vi "Nickname (Read).vi"(6 "ISOBUS address":T2=-1 caption="ISOBUS address (-1)", 8 "error in":errorcluster, 11 "Mercury Reference In":T3) -> (0 "error out":errorcluster, 2 "Nickname":string, 3 "Mercury Reference Out":T3, 4 "Valid?":T1)   [LabVIEW 2013, in "Mercury iXX.lvlib" / "Pressure.lvlib"]
doc: "Read the Nickname of the selected pressure device."
uses:
  <instrlib>/Mercury iXX/Public/Libraries/Pressure.lvlib
  <instrlib>/Mercury iXX/Public/Controls/Mercury Reference.ctl
  <instrlib>/Mercury iXX/Public/Controls/Comms Transport Layer.ctl
  <instrlib>/Mercury iXX/Private/Controls/Query Dynamic Reference.ctl
  <instrlib>/Mercury iXX/Public/Controls/ISOBus Address.ctl
  <instrlib>/Mercury iXX/Public/Controls/Is Valid LED.ctl
  <instrlib>/Mercury iXX/Private/Controls/Command Verbs.ctl
  <instrlib>/Mercury iXX/Mercury iXX.lvlib
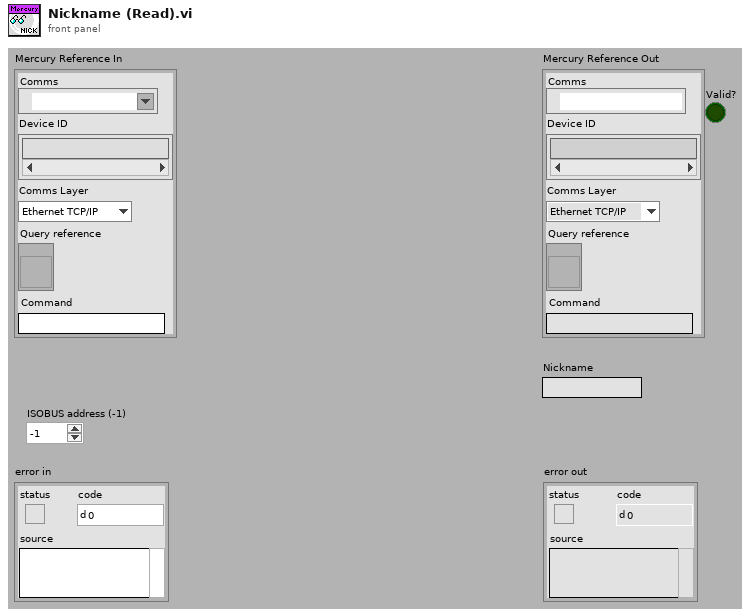
[diagram p1: front panel]
types:
  T1 = typedef "Mercury iXX.lvlib/Is Valid LED.ctl" = bool
  T2 = typedef "Mercury iXX.lvlib/ISOBus Address.ctl" = i32
  T3 = typedef "Mercury iXX.lvlib/Mercury Reference.ctl" = cluster{"Comms":refnum<visa-resource-name>, "Device ID":string[], "Comms Layer":T4, "Command":string, "Query reference":T5}
  T4 = typedef "Mercury iXX.lvlib/Comms Transport Layer.ctl" = enum16{"Ethernet TCP/IP", "USB", "ISOBus - RS-232", "GPIB"}
  T5 = typedef "Mercury iXX.lvlib/Query Dynamic Reference.ctl" = refnum<vi>
  T6 = typedef "Mercury iXX.lvlib/Command Verbs.ctl" = string
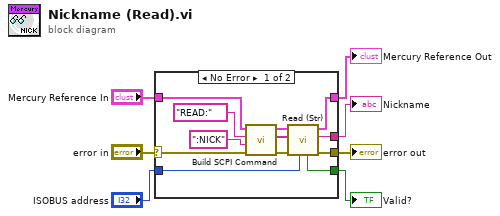
[diagram p0: block diagram]
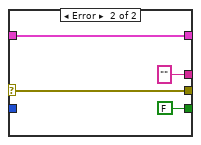
[diagram p2: hidden frame]
diagram:
  n1 = case shown="No Error" "error in" {
    selector: "error in" -> [w8 w23]
    tunnel: [w14 w22] -> w7
    tunnel: "Mercury Reference In" -> [w13 w22]
    tunnel: "ISOBUS address" -> [w12 _]
    tunnel: [w11 T1 FALSE ("Valid?")] -> w4
    tunnel: [w10 w23] -> w3
    tunnel: [w9 "" ("Response")] -> w2
    frame No Error {
      n2 = call <instrlib>:"Build SCPI Command.vi"("error in"=w8, "Noun(s)"=":NICK" ("Command"), "Verb"=T6 "READ:", "Mercury Reference In"=w13) -> ("error out"=w19:errorcluster, "SCPI Message(s)"=w16:string[], "Mercury Reference Out"=w17:T3)  [unwired: 5 out]
      n3 = call <instrlib>:"Read (Str).vi"("ISOBUS address"=w12, "error in"=w19, "SCPI Message(s)"=w16, "Mercury Reference In"=w17) -> ("error out"=w10:errorcluster, "Response"=w9:string, "Mercury Reference Out"=w14:T3, "Valid?"=w11:T1)  [unwired: 4 out]
    }
    frame Error {
    }
  }
  "Mercury Reference Out" <- w7
  "error out" <- w3
  "Nickname" <- w2
  "Valid?" <- w4
